vi "Hexapod_OLD_GUI.vi"() -> ()   [LabVIEW 2011]
panel:
  in  "z 2":dbl
  in  "y 2":dbl
  in  "x 2":dbl
  in  "z":dbl
  in  "y":dbl
  in  "x":dbl
  in  "M4StageNeg":bool
  in  "M4StagePos":bool
  in  "OAP1StageNeg":bool
  in  "OAP1StagePos":bool
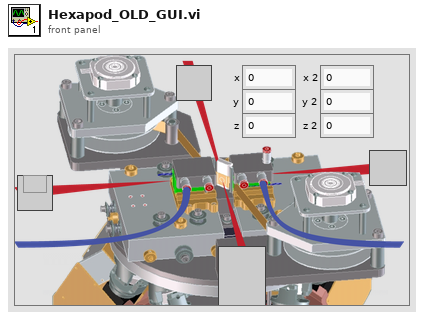
[diagram p1: front panel]
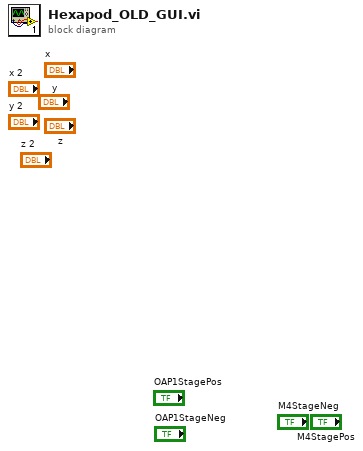
[diagram p0: block diagram]
diagram:
